vi "fgv_ROI ajustment codes.vi"(7 "FGV Actions":T1, 8 "error in (no error)":errorcluster, 10 "Z stop codes IN":u8[](array[numeric]), 11 "Z start codes IN":u8[](array[numeric])) -> (0 "error out":errorcluster, 2 "Z stop codes OUT":u8[](array[numeric]), 3 "Z start codes OUT":u8[](array[numeric]))   [LabVIEW 2017]
uses:
  Typedefs/fgv_actions.ctl
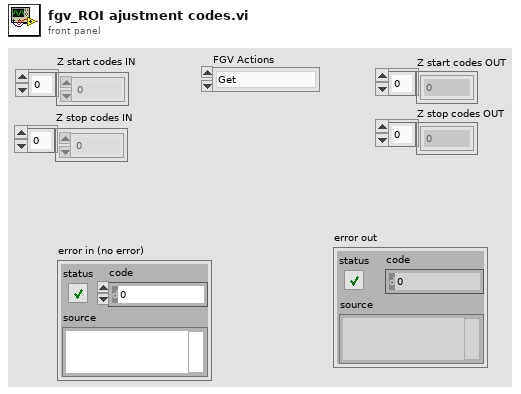
[diagram p1: front panel]
types:
  T1 = typedef "fgv_actions.ctl" = enum16{"Get", "Set"}
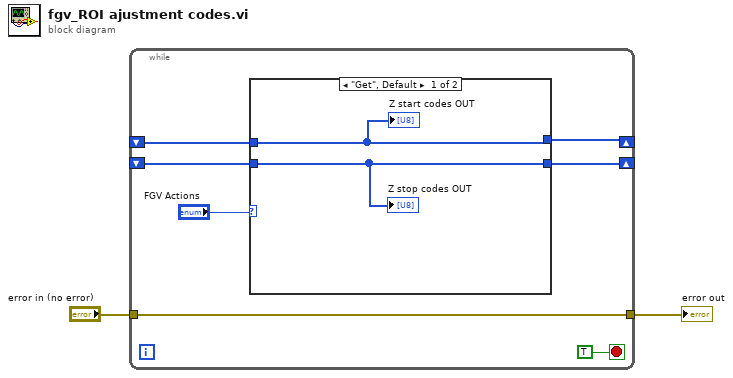
[diagram p0: block diagram]
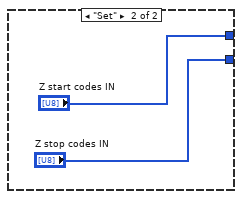
[diagram p2: hidden frame]
diagram:
  n1 = while {
    shift-right: [w7] -> _
    shift-left: _ -> [w6]
    shift-right: [w5] -> _
    shift-left: _ -> [w4]
    tunnel: "error in (no error)" -> [w3]
    tunnel: [w3] -> w1
    stop <- TRUE stop-if-true
    n2 = case shown="\"Get\", Default" "FGV Actions" {
      tunnel: [w11 "Z start codes IN"] -> w7
      tunnel: w6 -> [w11 _]
      tunnel: [w10 "Z stop codes IN"] -> w5
      tunnel: w4 -> [w10 _]
      frame "Get", Default {
        "Z start codes OUT" <- w11
        "Z stop codes OUT" <- w10
      }
      frame "Set" {
      }
    }
  }
  "error out" <- w1
